vi "Plotmatrix Scales Page.vi"() -> ()   [LabVIEW 2017, in "XY Plot Matrix.lvclass"]
uses:
  <vilib>/Math Plots/2D Math Plots/XY Plot Matrix/XY Plot Matrix/XY Plot Matrix.lvclass
  <vilib>/Math Plots/2D Math Plots/2D Plot/2D Plot/Typedef/Scale Array.ctl
  <vilib>/Math Plots/2D Math Plots/2D Plot/2D Plot/Typedef/Scale Cluster.ctl
  <vilib>/Utility/miscctls.llb/LVOffsetAndMultiplierTypeDef.ctl
  <vilib>/Math Plots/2D Math Plots/2D Plot/Action String/XYPlotMatrix Ctrl Act Queue.ctl
  <vilib>/Math Plots/2D Math Plots/2D Plot/Action String/XYPlotMatrix Ctrl Act Cluster.ctl
  <vilib>/Math Plots/2D Math Plots/2D Plot/Action String/2DMathPlot State Class.ctl
  <vilib>/Math Plots/2D Math Plots/2D Plot/2D Plot/Typedef/Dialog State.ctl
  <vilib>/Math Plots/2D Math Plots/2D Plot/2D Plot/Typedef/Temp Graph State.ctl
  <vilib>/Math Plots/2D Math Plots/2D Plot/2D Plot/Typedef/Temp Graph Property Action.ctl
  <vilib>/Math Plots/2D Math Plots/2D Plot/2D Plot/2D Plot.lvclass
panel:
  in  "Axis Name":string[](array[string])=["(X-Axis)", "(Y-Axis)"]
  in  "Event Registration":refnum<event-registration>
  in  "Control Ref Queue":T1
  out "Scale Array Out":T2
  in  "Scale Array In":T2
  in  "Current Scale":u16(ring) caption="Axes"
  in  "Multiplier":dbl
  in  "Offset":dbl
  in  "Scale Style":u16(ring) caption="Scale Style and Colors"
  in  "Grid Style":u16(ring) caption="Grid Style and Colors"
  in  "Show Scale Label":bool caption="Show scale label"
  in  "Maximum":dbl=10.0
  in  "Minimum":dbl
  in  "Minor Grid":u32(colorbox)=13056 caption="Minor grid"
  in  "Major Grid":u32(colorbox)=26112 caption="Major grid"
  in  "Marker Text":u32(colorbox) caption="Marker text"
  in  "Minor Tick":u32(colorbox) caption="Minor tick"
  in  "Major Tick":u32(colorbox) caption="Major tick"
  in  "Autoscale":bool
  in  "Log":bool
  in  "Show Scale":bool caption="Show scale"
  in  "Inverted":bool
  in  "Name":string
  # "Scaling Factors"
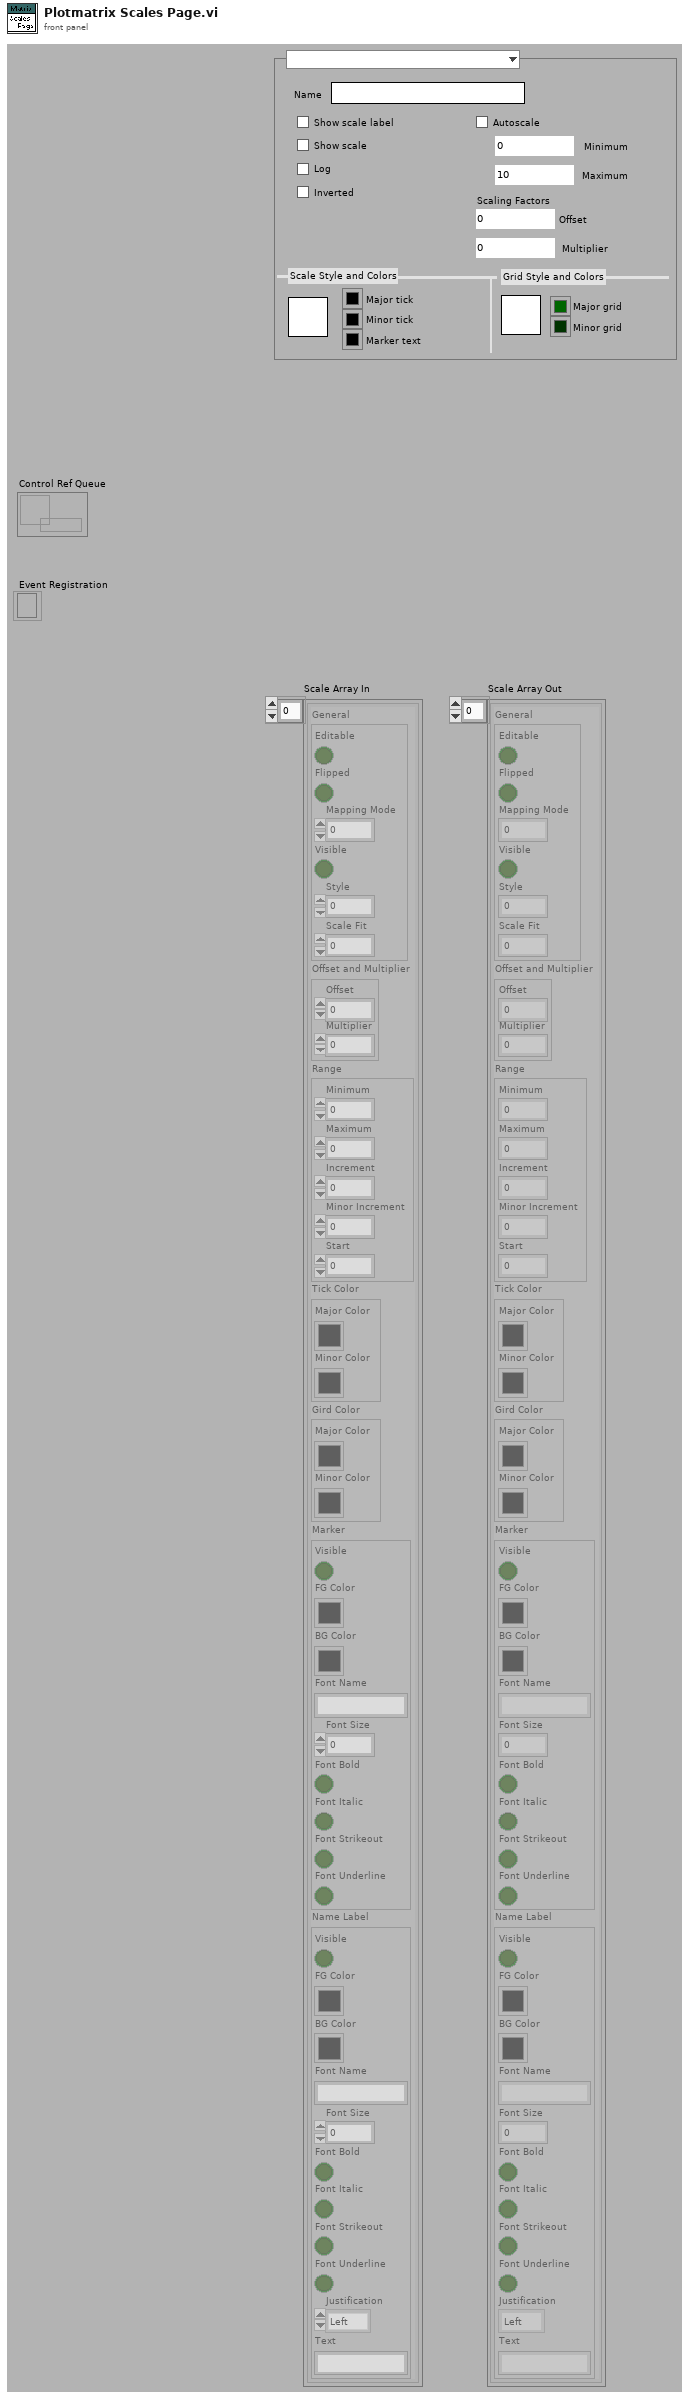
[diagram p1: front panel]
types:
  T1 = typedef "XYPlotMatrix Ctrl Act Queue.ctl" = refnum<queue>
  T2 = typedef "2D Plot.lvclass/Scale Array.ctl" = T3[]
  T3 = typedef "2D Plot.lvclass/Scale Cluster.ctl" = cluster{"General":cluster{"Editable":bool, "Flipped":bool, "Mapping Mode":u8, "Visible":bool, "Style":u8, "Scale Fit":u8}, "Offset and Multiplier":T4, "Range":cluster{"Minimum":dbl, "Maximum":dbl, "Increment":dbl, "Minor Increment":dbl, "Start":dbl}, "Tick Color":cluster{"Major Color":u32, "Minor Color":u32}, "Gird Color":cluster{"Major Color":u32, "Minor Color":u32}, "Marker":cluster{"Visible":bool, "FG Color":u32, "BG Color":u32, "Font Name":string, "Font Size":u32, "Font Bold":bool, "Font Italic":bool, "Font Strikeout":bool, "Font Underline":bool}, "Name Label":cluster{"Visible":bool, "FG Color":u32, "BG Color":u32, "Font Name":string, "Font Size":u32, "Font Bold":bool, "Font Italic":bool, "Font Strikeout":bool, "Font Underline":bool, "Justification":enum16{"Left", "Center", "Right"}, "Text":string}}
  T4 = typedef "LVOffsetAndMultiplierTypeDef.ctl" = cluster{"Offset":dbl, "Multiplier":dbl}
  T5 = typedef "2D Plot.lvclass/Dialog State.ctl" = enum16{"Initialize", "Read Property", "Write Property", "Idle", "Exit"}
  T6 = typedef "2D Plot.lvclass/Temp Graph Property Action.ctl" = enum16{"Appearance Property", "Format Property", "Plots Property", "Scales Property"}
  T7 = typedef "2D Plot.lvclass/Temp Graph State.ctl" = enum16{"Create", "Update Graph", "Update Property Only", "Get Plot Name", "Get Axis Name", "Destory"}
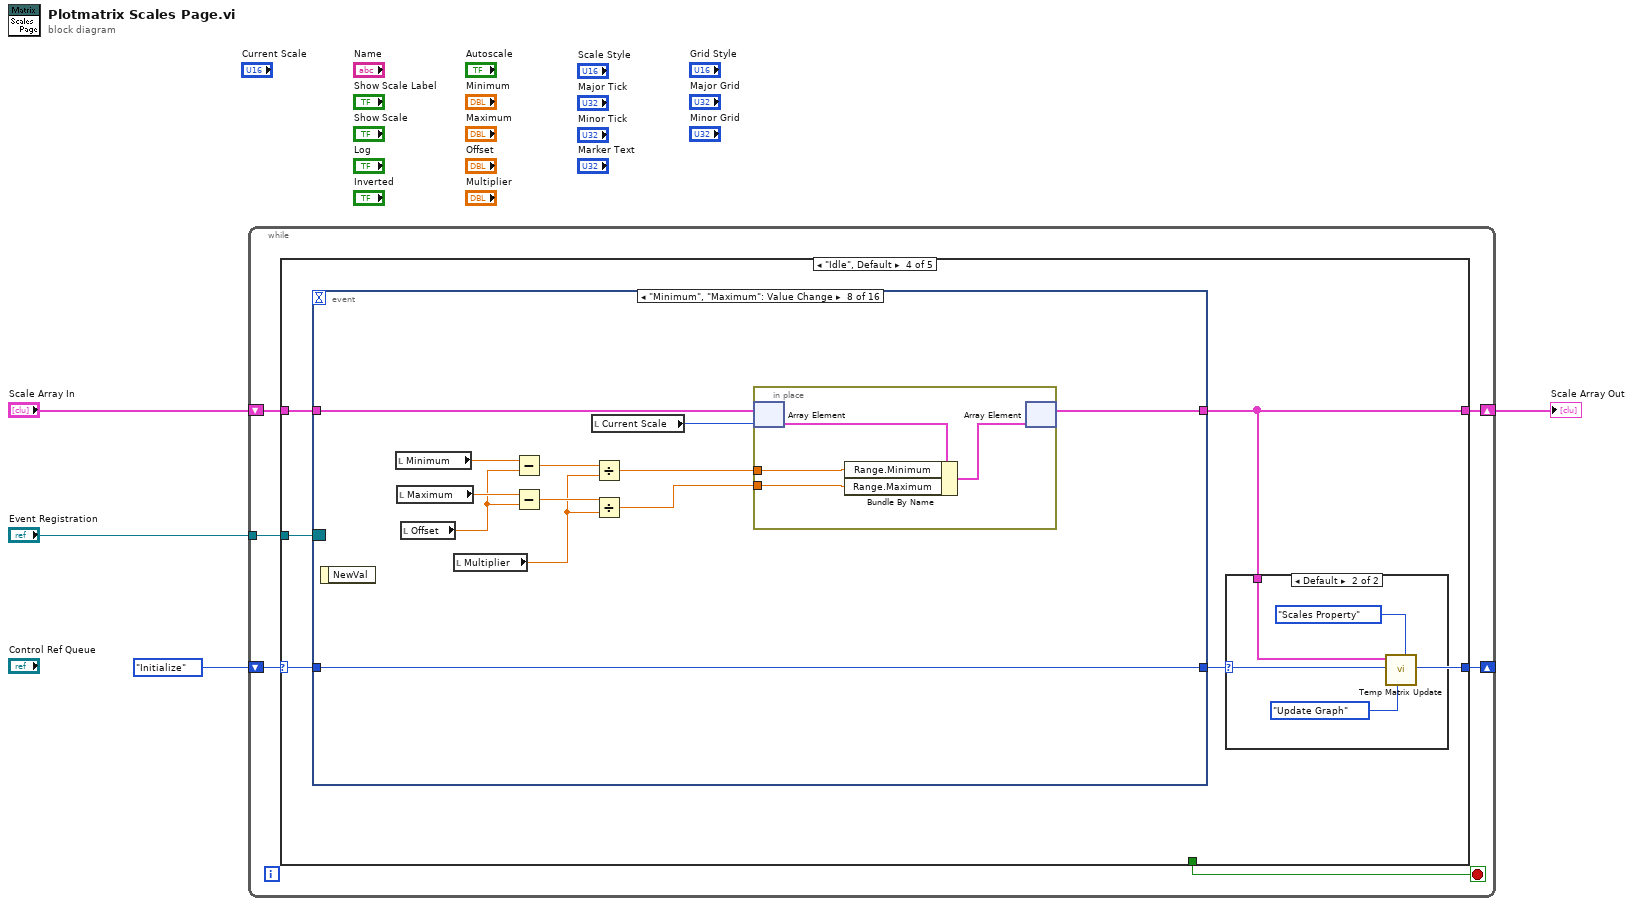
[diagram p0: block diagram]
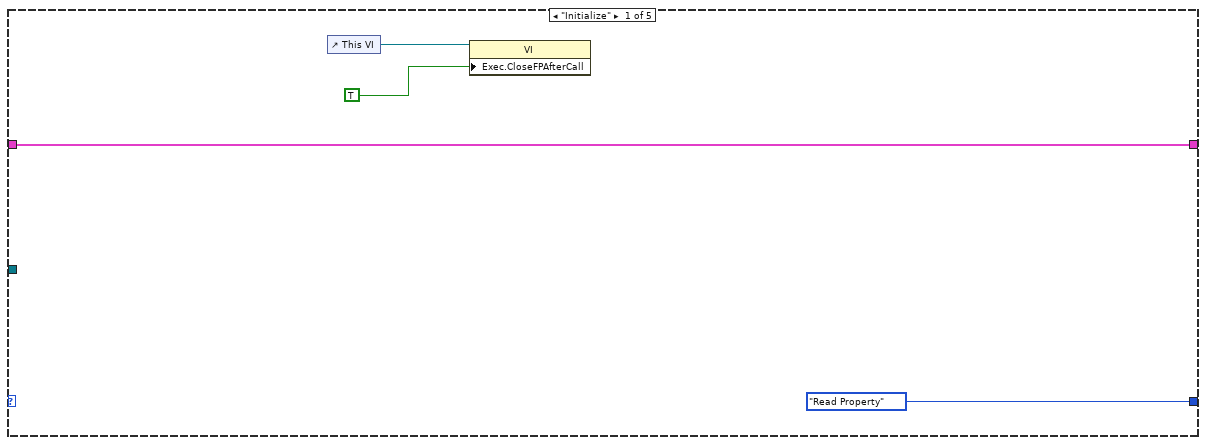
[diagram p2: hidden frame]
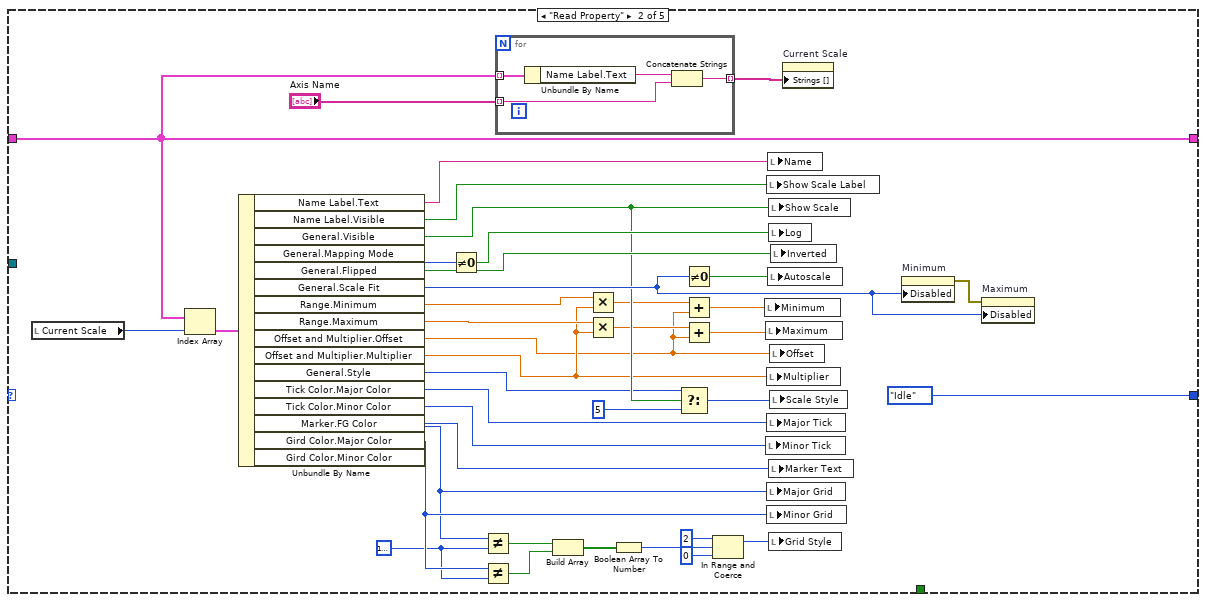
[diagram p3: hidden frame]
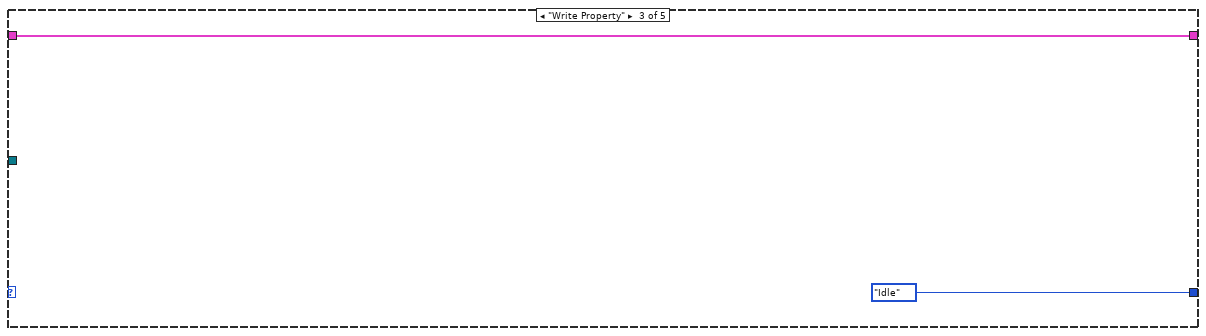
[diagram p4: hidden frame]
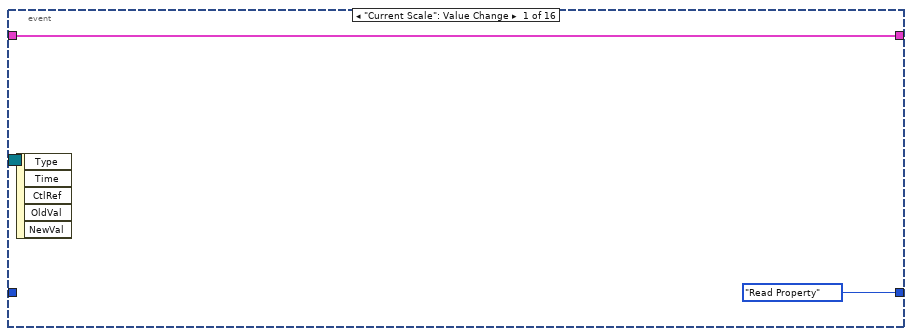
[diagram p6: hidden frame]
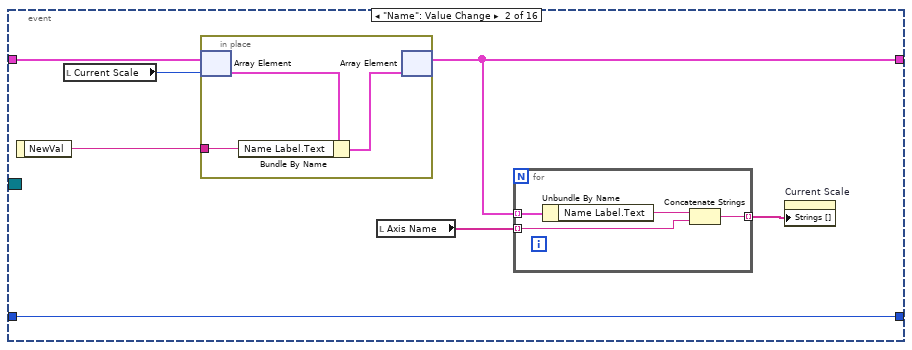
[diagram p7: hidden frame]
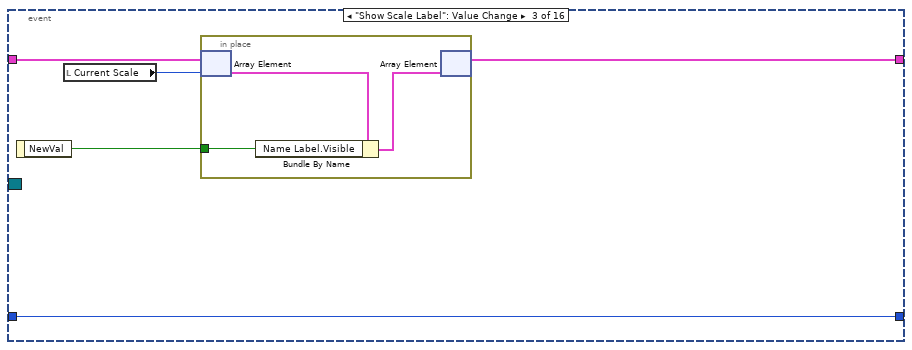
[diagram p8: hidden frame]
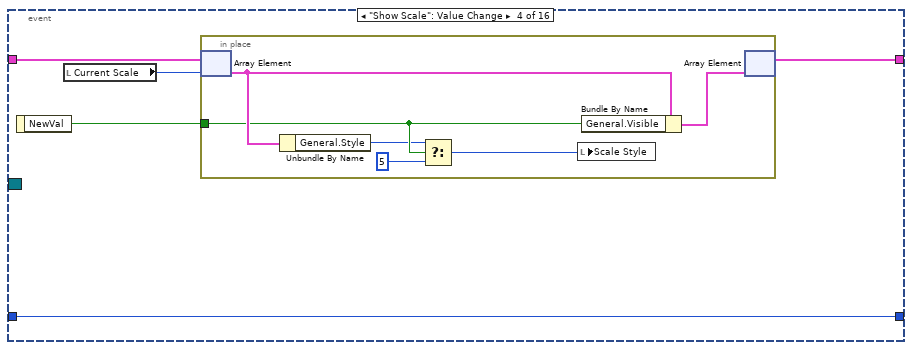
[diagram p9: hidden frame]
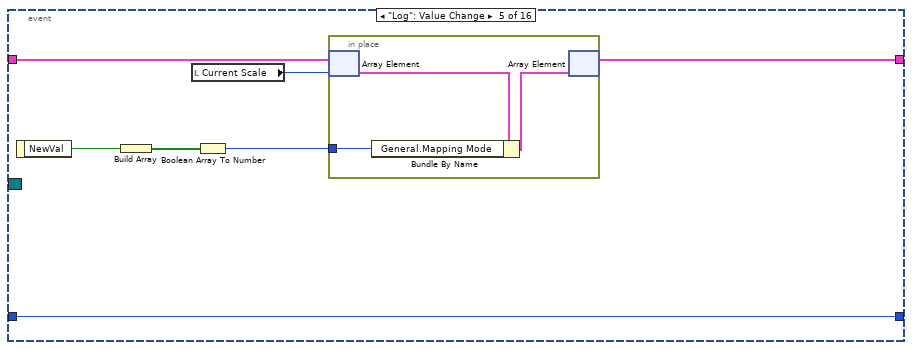
[diagram p10: hidden frame]
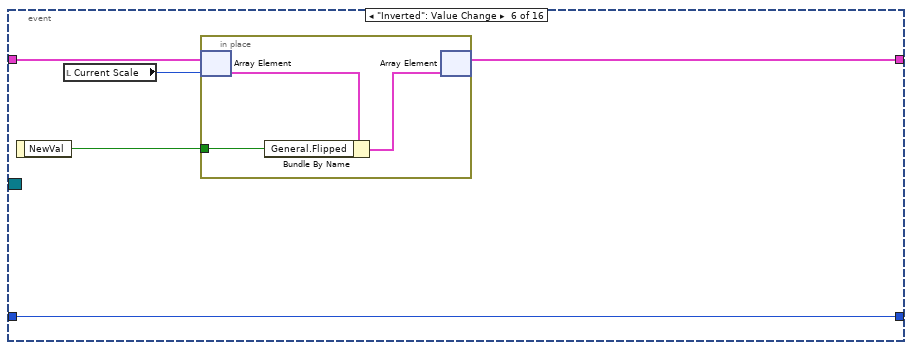
[diagram p11: hidden frame]
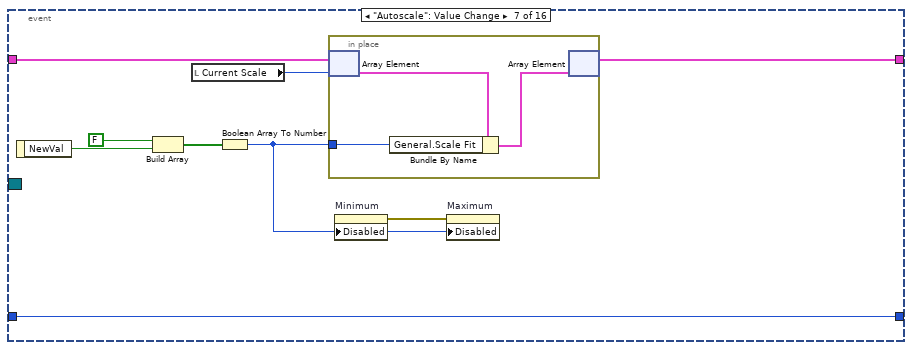
[diagram p12: hidden frame]
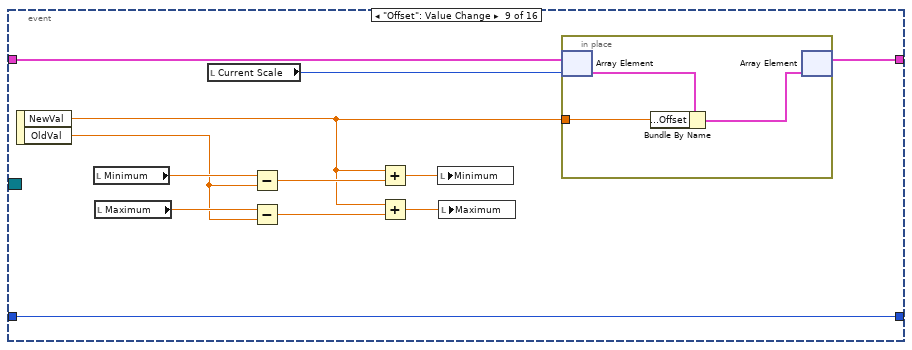
[diagram p13: hidden frame]
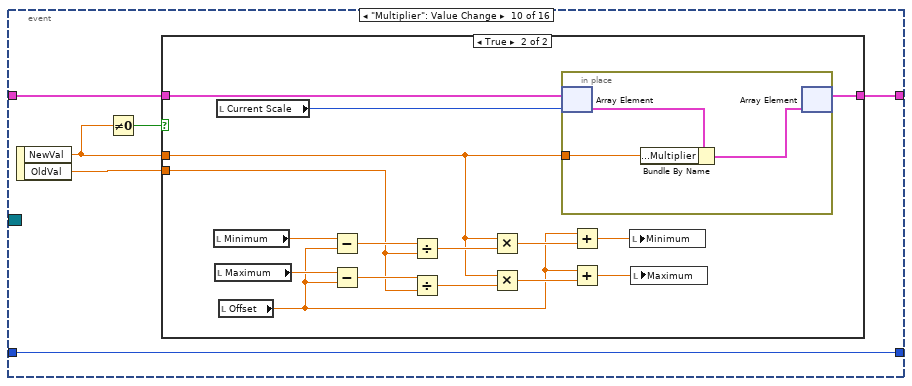
[diagram p14: hidden frame]
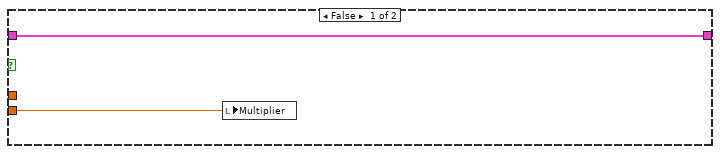
[diagram p15: hidden frame]
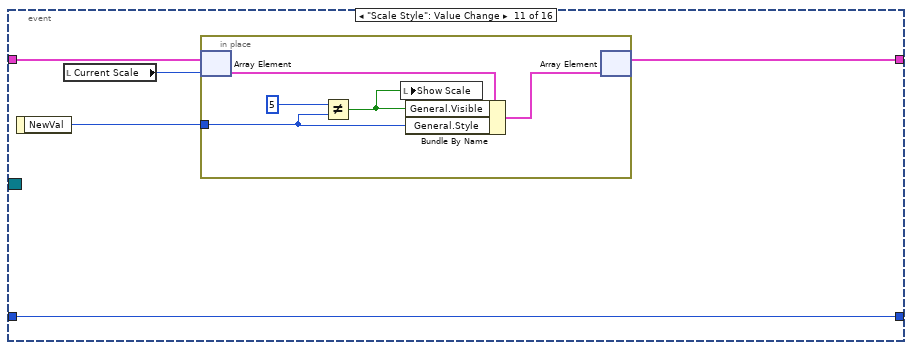
[diagram p16: hidden frame]
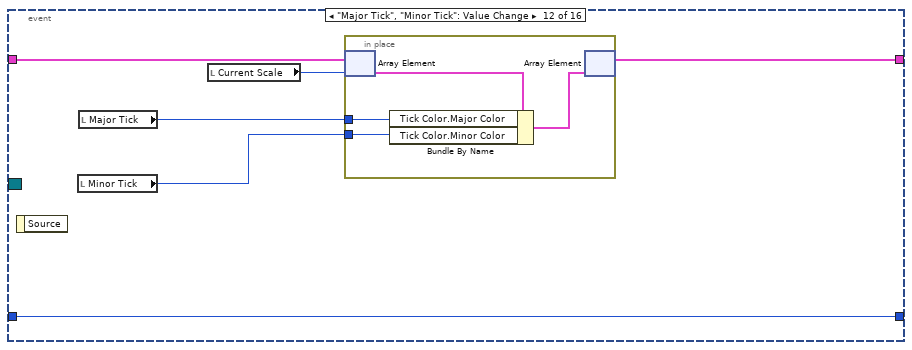
[diagram p17: hidden frame]
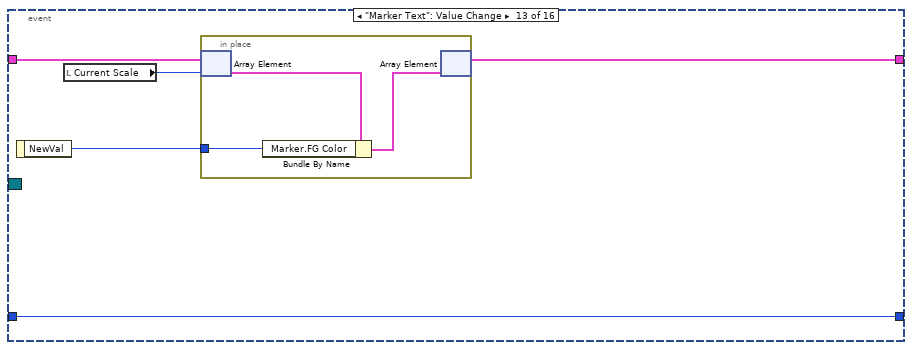
[diagram p18: hidden frame]
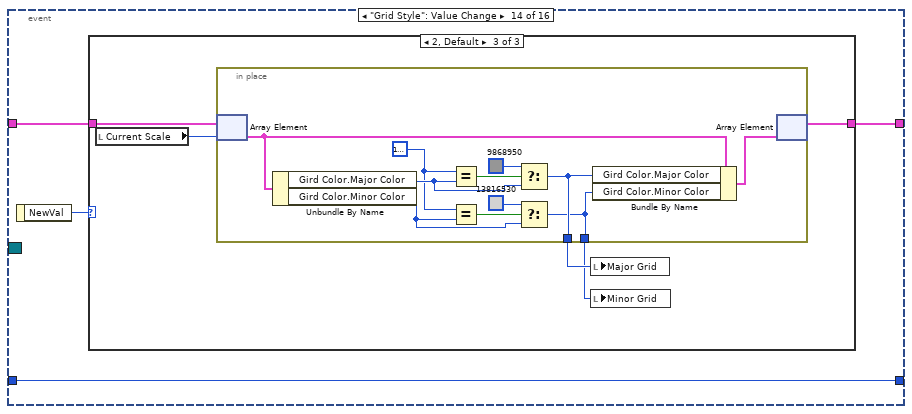
[diagram p19: hidden frame]
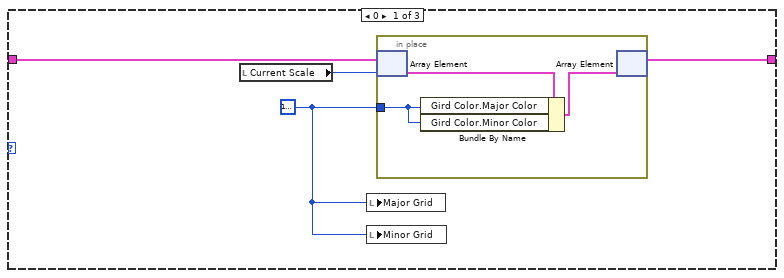
[diagram p20: hidden frame]
diagram:
  n1 = while {
    shift-right: [w7] -> _
    shift-left: Dialog_State."Initialize" ("Enum") -> [w10]
    shift-right: [w8] -> w3
    shift-left: "Scale Array In" -> [w9]
    tunnel: "Event Registration" -> [w5]
    stop <- w6 stop-if-true
    n2 = case shown="\"Idle\", Default" w10 {
      selector: w10 -> [_ _ _ w62 w280]
      tunnel: w9 -> [w12 w32 w59 w64 w278]
      tunnel: [w12 w32 w59 w61 w278] -> w8
      tunnel: [Dialog_State."Read Property" ("Enum") Dialog_State."Idle" ("Enum") Dialog_State."Idle" ("Enum") w60 w280] -> w7
      tunnel: [_ _ _ _ TRUE] -> w6
      tunnel: w5 -> [_ _ _ w63 _]
      frame "Initialize" {
        n3 = control-ref of="This VI"() -> (w14:refnum<vi>)
        n4 = property class="VI"(reference=w14, "Exec.CloseFPAfterCall"=TRUE ("Execution:Close After Call")) -> ()  [unwired: 1 in, 2 out]
      }
      frame "Read Property" {
        w34 = u32 16777216
        n5 = local read "Current Scale"() -> (w53:u16)
        n6 = Index Array(array=w32, index=w53) -> (element=w52:T3)
        n7 = Unbundle By Name(w52) -> ("Name Label.Text"=w51:string, "Name Label.Visible"=w50:bool, "General.Visible"=w26:bool, "General.Mapping Mode"=w49:u8, "General.Flipped"=w47:bool, "General.Scale Fit"=w45:u8, "Range.Minimum"=w22:dbl, "Range.Maximum"=w20:dbl, "Offset and Multiplier.Offset"=w17:dbl, "Offset and Multiplier.Multiplier"=w19:dbl, "General.Style"=w25:u8, "Tick Color.Major Color"=w43:u32, "Tick Color.Minor Color"=w41:u32, "Marker.FG Color"=w42:u32, "Gird Color.Major Color"=w38:u32, "Gird Color.Minor Color"=w39:u32)
        n8 = Not Equal To 0?(x=w49) -> (x != 0?=w48:bool)
        n9 = Not Equal?(x=w38, y=w34) -> (x != y?=w36:bool)
        n10 = Not Equal?(x=w39, y=w34) -> (x != y?=w37:bool)
        n11 = for {
          tunnel: w32 -> [w57] mode=indexing
          tunnel: "Axis Name" -> [w55] mode=indexing
          tunnel: [w54] -> w33 mode=indexing
          n12 = Unbundle By Name(w57) -> ("Name Label.Text"=w56:string)
          n13 = Concatenate Strings(w56, w55) -> (w54:string)
        }
        n14 = Build Array(w36, w37) -> (w35:bool[])
        n15 = Multiply(x=w22, y=w19) -> (x*y=w21:dbl)
        n16 = Multiply(x=w20, y=w19) -> (x*y=w18:dbl)
        n17 = Boolean Array To Number(Boolean array=w35) -> (number=w30:u16)
        n18 = Select(t=w25, s=w26, f=u8 5) -> (s? t:f=w23:u8)
        n19 = Not Equal To 0?(x=w45) -> (x != 0?=w46:bool)
        n20 = Add(x=w21, y=w17) -> (x+y=w16:dbl)
        n21 = Add(x=w18, y=w17) -> (x+y=w15:dbl)
        n22 = In Range and Coerce(upper limit=u16 2, x=w30, lower limit=u16 0) -> (coerced(x)=w27:u16)  [unwired: 1 out]
        n23 = local write "Minimum"(w16) -> ()
        n24 = local write "Maximum"(w15) -> ()
        n25 = local write "Minor Tick"(w41) -> ()
        n26 = local write "Show Scale Label"(w50) -> ()
        n27 = local write "Multiplier"(w19) -> ()
        n28 = local write "Major Tick"(w43) -> ()
        n29 = local write "Major Grid"(w38) -> ()
        n30 = local write "Minor Grid"(w39) -> ()
        n31 = local write "Name"(w51) -> ()
        n32 = local write "Autoscale"(w46) -> ()
        n33 = local write "Show Scale"(w26) -> ()
        n34 = local write "Log"(w48) -> ()
        n35 = local write "Marker Text"(w42) -> ()
        n36 = local write "Grid Style"(w27) -> ()
        n37 = local write "Offset"(w17) -> ()
        n38 = local write "Scale Style"(w23) -> ()
        n39 = local write "Inverted"(w47) -> ()
        n40 = property on="Current Scale" class="Ring (strict)"("Strings []"=w33) -> ()  [unwired: 2 in, 2 out]
        n41 = property on="Minimum" class="DigNum (strict)"("Disabled"=w45) -> (error out=w40:errorcluster)  [unwired: 2 in, 1 out]
        n42 = property on="Maximum" class="DigNum (strict)"(error in=w40, "Disabled"=w45) -> ()  [unwired: 1 in, 2 out]
      }
      frame "Write Property" {
      }
      frame "Idle", Default {
        n43 = event shown="[7] \"Minimum\", \"Maximum\": Value Change" {
          selector: w63 -> [_ _ _ _ _ _ _ _ _ _ _ _ _ _ _ _]
          dyn-events: _ -> [_ _ _ _ _ _ _ _ _ _ _ _ _ _ _ _]
          timeout: _ -> [_ _ _ _ _ _ _ _ _ _ _ _ _ _ _ _]
          tunnel: w64 -> [w69 w76 w88 w96 w109 w117 w129 w144 w160 w169 w195 w206 w215 w222 w271 w277]
          tunnel: [w69 w74 w87 w95 w108 w116 w128 w143 w159 w168 w194 w205 w214 w221 w270 w277] -> w61
          tunnel: [Dialog_State."Read Property" ("Enum") w71 w84 w92 w103 w113 w122 w141 w158 w166 w192 w201 w211 w219 w262 Dialog_State."Exit" ("Enum")] -> w60
          tunnel: w62 -> [_ w71 w84 w92 w103 w113 w122 w141 w158 w166 w192 w201 w211 w219 w262 _]
          event "Current Scale": Value Change {
            n44 = event-data() -> ()  [unwired: 6 out]
          }
          event "Name": Value Change {
            n45 = event-data() -> ("NewVal"=w72:string)  [unwired: 1 out]
            n46 = local read "Current Scale"() -> (w73:u16)
            n47 = in-place {
              in-place-border: w72 -> [w81]
              n48 = in-place-array #1(w76, w73) -> (w83:T3)
              n49 = Bundle By Name(cluster=w83, "Name Label.Text"=w81) -> (w82:T3)
              n50 = in-place-array #1(w82) -> (w74:T2)  [unwired: 1 out]
            }
            n51 = local read "Axis Name"() -> (w70:string[])
            n52 = for {
              tunnel: w74 -> [w80] mode=indexing
              tunnel: w70 -> [w78] mode=indexing
              tunnel: [w77] -> w75 mode=indexing
              n53 = Unbundle By Name(w80) -> ("Name Label.Text"=w79:string)
              n54 = Concatenate Strings(w79, w78) -> (w77:string)
            }
            n55 = property on="Current Scale" class="Ring (strict)"("Strings []"=w75) -> ()  [unwired: 2 in, 2 out]
          }
          event "Show Scale Label": Value Change {
            n56 = event-data() -> ("NewVal"=w85:bool)  [unwired: 1 out]
            n57 = local read "Current Scale"() -> (w86:u16)
            n58 = in-place {
              in-place-border: w85 -> [w89]
              n59 = in-place-array #2(w88, w86) -> (w91:T3)
              n60 = Bundle By Name(cluster=w91, "Name Label.Visible"=w89) -> (w90:T3)
              n61 = in-place-array #2(w90) -> (w87:T2)  [unwired: 1 out]
            }
          }
          event "Show Scale": Value Change {
            n62 = event-data() -> ("NewVal"=w93:bool)  [unwired: 1 out]
            n63 = local read "Current Scale"() -> (w94:u16)
            n64 = in-place {
              in-place-border: w93 -> [w99]
              n65 = in-place-array #3(w96, w94) -> (w101:T3)
              n66 = Unbundle By Name(w101) -> ("General.Style"=w98:u8)
              n67 = Select(t=w98, s=w99, f=u8 5) -> (s? t:f=w97:u8)
              n68 = local write "Scale Style"(w97) -> ()
              n69 = Bundle By Name(cluster=w101, "General.Visible"=w99) -> (w102:T3)
              n70 = in-place-array #3(w102) -> (w95:T2)  [unwired: 1 out]
            }
          }
          event "Log": Value Change {
            n71 = event-data() -> ("NewVal"=w106:bool)  [unwired: 1 out]
            n72 = Build Array(w106) -> (w105:bool[])
            n73 = local read "Current Scale"() -> (w107:u16)
            n74 = Boolean Array To Number(Boolean array=w105) -> (number=w104:u8)
            n75 = in-place {
              in-place-border: w104 -> [w110]
              n76 = in-place-array #4(w109, w107) -> (w112:T3)
              n77 = Bundle By Name(cluster=w112, "General.Mapping Mode"=w110) -> (w111:T3)
              n78 = in-place-array #4(w111) -> (w108:T2)  [unwired: 1 out]
            }
          }
          event "Inverted": Value Change {
            n79 = event-data() -> ("NewVal"=w114:bool)  [unwired: 1 out]
            n80 = local read "Current Scale"() -> (w115:u16)
            n81 = in-place {
              in-place-border: w114 -> [w118]
              n82 = in-place-array #5(w117, w115) -> (w120:T3)
              n83 = Bundle By Name(cluster=w120, "General.Flipped"=w118) -> (w119:T3)
              n84 = in-place-array #5(w119) -> (w116:T2)  [unwired: 1 out]
            }
          }
          event "Autoscale": Value Change {
            n85 = event-data() -> ("NewVal"=w126:bool)  [unwired: 1 out]
            n86 = Build Array(FALSE ("element"), w126) -> (w125:bool[])
            n87 = local read "Current Scale"() -> (w127:u16)
            n88 = Boolean Array To Number(Boolean array=w125) -> (number=w123:u8)
            n89 = in-place {
              in-place-border: w123 -> [w130]
              n90 = in-place-array #6(w129, w127) -> (w132:T3)
              n91 = Bundle By Name(cluster=w132, "General.Scale Fit"=w130) -> (w131:T3)
              n92 = in-place-array #6(w131) -> (w128:T2)  [unwired: 1 out]
            }
            n93 = property on="Minimum" class="DigNum (strict)"("Disabled"=w123) -> (error out=w124:errorcluster)  [unwired: 2 in, 1 out]
            n94 = property on="Maximum" class="DigNum (strict)"(error in=w124, "Disabled"=w123) -> ()  [unwired: 1 in, 2 out]
          }
          event "Minimum", "Maximum": Value Change {
            n95 = event-data() -> ()  [unwired: 2 out]
            n96 = local read "Minimum"() -> (w138:dbl)
            n97 = local read "Maximum"() -> (w137:dbl)
            n98 = local read "Offset"() -> (w136:dbl)
            n99 = local read "Multiplier"() -> (w135:dbl)
            n100 = Subtract(x=w138, y=w136) -> (x-y=w140:dbl)
            n101 = Subtract(x=w137, y=w136) -> (x-y=w139:dbl)
            n102 = local read "Current Scale"() -> (w142:u16)
            n103 = Divide(x=w140, y=w135) -> (x/y=w134:dbl)
            n104 = Divide(x=w139, y=w135) -> (x/y=w133:dbl)
            n105 = in-place {
              in-place-border: w134 -> [w146]
              in-place-border: w133 -> [w145]
              n106 = in-place-array #7(w144, w142) -> (w148:T3)
              n107 = Bundle By Name(cluster=w148, "Range.Minimum"=w146, "Range.Maximum"=w145) -> (w147:T3)
              n108 = in-place-array #7(w147) -> (w143:T2)  [unwired: 1 out]
            }
          }
          event "Offset": Value Change {
            n109 = event-data() -> ("NewVal"=w149:dbl, "OldVal"=w153:dbl)  [unwired: 1 out]
            n110 = local read "Minimum"() -> (w155:dbl)
            n111 = local read "Maximum"() -> (w154:dbl)
            n112 = local read "Current Scale"() -> (w152:u16)
            n113 = Subtract(x=w155, y=w153) -> (x-y=w156:dbl)
            n114 = Subtract(x=w154, y=w153) -> (x-y=w157:dbl)
            n115 = Add(x=w149, y=w156) -> (x+y=w151:dbl)
            n116 = Add(x=w149, y=w157) -> (x+y=w150:dbl)
            n117 = local write "Minimum"(w151) -> ()
            n118 = local write "Maximum"(w150) -> ()
            n119 = in-place {
              in-place-border: w149 -> [w161]
              n120 = in-place-array #8(w160, w152) -> (w163:T3)
              n121 = Bundle By Name(cluster=w163, "Offset and Multiplier.Offset"=w161) -> (w162:T3)
              n122 = in-place-array #8(w162) -> (w159:T2)  [unwired: 1 out]
            }
          }
          event "Multiplier": Value Change {
            n123 = event-data() -> ("NewVal"=w165:dbl, "OldVal"=w167:dbl)  [unwired: 1 out]
            n124 = Not Equal To 0?(x=w165) -> (x != 0?=w164:bool)
            n125 = case shown="True" w164 {
              tunnel: w169 -> [w170 w187]
              tunnel: [w170 w186] -> w168
              tunnel: w167 -> [w171 w175]
              tunnel: w165 -> [_ w172]
              frame False {
                n126 = local write "Multiplier"(w171) -> ()
              }
              frame True {
                n127 = local read "Minimum"() -> (w178:dbl)
                n128 = local read "Maximum"() -> (w177:dbl)
                n129 = local read "Current Scale"() -> (w179:u16)
                n130 = local read "Offset"() -> (w176:dbl)
                n131 = Subtract(x=w178, y=w176) -> (x-y=w183:dbl)
                n132 = Subtract(x=w177, y=w176) -> (x-y=w182:dbl)
                n133 = Divide(x=w183, y=w175) -> (x/y=w184:dbl)
                n134 = Divide(x=w182, y=w175) -> (x/y=w185:dbl)
                n135 = Multiply(x=w172, y=w184) -> (x*y=w180:dbl)
                n136 = Multiply(x=w172, y=w185) -> (x*y=w181:dbl)
                n137 = in-place {
                  in-place-border: w172 -> [w188]
                  n138 = in-place-array #9(w187, w179) -> (w190:T3)
                  n139 = Bundle By Name(cluster=w190, "Offset and Multiplier.Multiplier"=w188) -> (w189:T3)
                  n140 = in-place-array #9(w189) -> (w186:T2)  [unwired: 1 out]
                }
                n141 = Add(x=w176, y=w180) -> (x+y=w174:dbl)
                n142 = Add(x=w176, y=w181) -> (x+y=w173:dbl)
                n143 = local write "Minimum"(w174) -> ()
                n144 = local write "Maximum"(w173) -> ()
              }
            }
          }
          event "Scale Style": Value Change {
            n145 = event-data() -> ("NewVal"=w193:u16)  [unwired: 1 out]
            n146 = local read "Current Scale"() -> (w191:u16)
            n147 = in-place {
              in-place-border: w193 -> [w198]
              n148 = in-place-array #10(w195, w191) -> (w200:T3)
              n149 = Not Equal?(x=u16 5, y=w198) -> (x != y?=w196:bool)
              n150 = local write "Show Scale"(w196) -> ()
              n151 = Bundle By Name(cluster=w200, "General.Visible"=w196, "General.Style"=w198) -> (w199:T3)
              n152 = in-place-array #10(w199) -> (w194:T2)  [unwired: 1 out]
            }
          }
          event "Major Tick", "Minor Tick": Value Change {
            n153 = event-data() -> ()  [unwired: 2 out]
            n154 = local read "Minor Tick"() -> (w202:u32)
            n155 = local read "Major Tick"() -> (w203:u32)
            n156 = local read "Current Scale"() -> (w204:u16)
            n157 = in-place {
              in-place-border: w203 -> [w208]
              in-place-border: w202 -> [w207]
              n158 = in-place-array #11(w206, w204) -> (w210:T3)
              n159 = Bundle By Name(cluster=w210, "Tick Color.Major Color"=w208, "Tick Color.Minor Color"=w207) -> (w209:T3)
              n160 = in-place-array #11(w209) -> (w205:T2)  [unwired: 1 out]
            }
          }
          event "Marker Text": Value Change {
            n161 = event-data() -> ("NewVal"=w212:u32)  [unwired: 1 out]
            n162 = local read "Current Scale"() -> (w213:u16)
            n163 = in-place {
              in-place-border: w212 -> [w216]
              n164 = in-place-array #12(w215, w213) -> (w218:T3)
              n165 = Bundle By Name(cluster=w218, "Marker.FG Color"=w216) -> (w217:T3)
              n166 = in-place-array #12(w217) -> (w214:T2)  [unwired: 1 out]
            }
          }
          event "Grid Style": Value Change {
            n167 = event-data() -> ("NewVal"=w220:u16)  [unwired: 1 out]
            n168 = case shown="2, Default" w220 {
              tunnel: w222 -> [w226 w234 w246]
              tunnel: [w225 w233 w245] -> w221
              frame 0 {
                w223 = u32 16777216
                n169 = local read "Current Scale"() -> (w224:u16)
                n170 = local write "Major Grid"(w223) -> ()
                n171 = local write "Minor Grid"(w223) -> ()
                n172 = in-place {
                  in-place-border: w223 -> [w227]
                  n173 = in-place-array #13(w226, w224) -> (w229:T3)
                  n174 = Bundle By Name(cluster=w229, "Gird Color.Major Color"=w227, "Gird Color.Minor Color"=w227) -> (w228:T3)
                  n175 = in-place-array #13(w228) -> (w225:T2)  [unwired: 1 out]
                }
              }
              frame 1 {
                w230 = u32 16777216
                n176 = local read "Current Scale"() -> (w232:u16)
                n177 = in-place {
                  in-place-border: w230 -> [w239]
                  in-place-border: [w235] -> w231
                  n178 = in-place-array #14(w234, w232) -> (w240:T3)
                  n179 = Unbundle By Name(w240) -> ("Gird Color.Major Color"=w236:u32)
                  n180 = Equal?(x=w239, y=w236) -> (x = y?=w238:bool)
                  n181 = Select(t=u32 9868950 ("Major Grid"), s=w238, f=w236) -> (s? t:f=w235:u32)
                  n182 = Bundle By Name(cluster=w240, "Gird Color.Minor Color"=w239, "Gird Color.Major Color"=w235) -> (w241:T3)
                  n183 = in-place-array #14(w241) -> (w233:T2)  [unwired: 1 out]
                }
                n184 = local write "Major Grid"(w231) -> ()
                n185 = local write "Minor Grid"(w230) -> ()
              }
              frame 2, Default {
                n186 = local read "Current Scale"() -> (w244:u16)
                n187 = in-place {
                  in-place-border: [w252] -> w243
                  in-place-border: [w249] -> w242
                  w248 = u32 16777216
                  n188 = in-place-array #15(w246, w244) -> (w256:T3)
                  n189 = Unbundle By Name(w256) -> ("Gird Color.Major Color"=w253:u32, "Gird Color.Minor Color"=w247:u32)
                  n190 = Equal?(x=w248, y=w253) -> (x = y?=w255:bool)
                  n191 = Equal?(x=w248, y=w247) -> (x = y?=w251:bool)
                  n192 = Select(t=u32 9868950 ("Major Grid"), s=w255, f=w253) -> (s? t:f=w252:u32)
                  n193 = Select(t=u32 13816530 ("Minor Grid"), s=w251, f=w247) -> (s? t:f=w249:u32)
                  n194 = Bundle By Name(cluster=w256, "Gird Color.Major Color"=w252, "Gird Color.Minor Color"=w249) -> (w257:T3)
                  n195 = in-place-array #15(w257) -> (w245:T2)  [unwired: 1 out]
                }
                n196 = local write "Major Grid"(w243) -> ()
                n197 = local write "Minor Grid"(w242) -> ()
              }
            }
          }
          event "Major Grid", "Minor Grid": Value Change {
            w265 = u32 16777216
            n198 = event-data() -> ()  [unwired: 2 out]
            n199 = local read "Major Grid"() -> (w264:u32)
            n200 = local read "Minor Grid"() -> (w263:u32)
            n201 = local read "Current Scale"() -> (w269:u16)
            n202 = Not Equal?(x=w264, y=w265) -> (x != y?=w267:bool)
            n203 = Not Equal?(x=w263, y=w265) -> (x != y?=w268:bool)
            n204 = in-place {
              in-place-border: w264 -> [w273]
              in-place-border: w263 -> [w272]
              n205 = in-place-array #16(w271, w269) -> (w275:T3)
              n206 = Bundle By Name(cluster=w275, "Gird Color.Major Color"=w273, "Gird Color.Minor Color"=w272) -> (w274:T3)
              n207 = in-place-array #16(w274) -> (w270:T2)  [unwired: 1 out]
            }
            n208 = Build Array(w267, w268) -> (w266:bool[])
            n209 = Boolean Array To Number(Boolean array=w266) -> (number=w259:u16)
            n210 = In Range and Coerce(upper limit=u16 2, x=w259, lower limit=u16 0) -> (coerced(x)=w258:u16)  [unwired: 1 out]
            n211 = local write "Grid Style"(w258) -> ()
          }
          event User Event {
            n212 = event-data() -> ()  [unwired: 6 out]
          }
        }
        n213 = case shown="Default" w60 {
          tunnel: w61 -> [_ w65]
          frame "Exit" {
          }
          frame Default {
            n214 = call <vilib>:"Temp Matrix Update.vi"("Property Name"=Temp_Graph_Property_Action."Scales Property", "State"=Temp_Graph_State."Update Graph", "Property In"=w65) -> ()  [unwired: 2 in, 7 out]
          }
        }
      }
      frame "Exit" {
      }
    }
  }
  "Scale Array Out" <- w3
